vi "Do.vi"(8 "error in (no error)":errorcluster, 10 "Actor in":refnum<class "Actor.lvclass">, 11 "Update Fan Status Msg":refnum<class "Update Fan Status Msg.lvclass">) -> (0 "error out":errorcluster, 2 "Actor out":refnum<class "Actor.lvclass">)   [LabVIEW 2018, in "Evaporative Cooler Controller.lvlib" / "Update Fan Status Msg.lvclass"]
uses:
  Update Fan Status Msg.lvclass
  <vilib>/ActorFramework/Actor/Actor.lvclass
  Evaporative Cooler Controller/Evaporative Cooler Controller.lvclass
  C:/Program Files (x86)/National Instruments/LabVIEW 2018/vi.lib/ActorFramework/Actor/Actor.lvclass
  Update Fan Status Msg.lvclass/Update Fan Status Msg.ctl
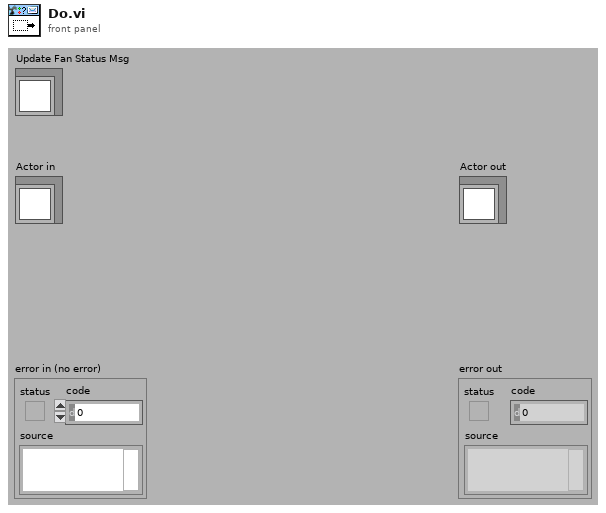
[diagram p1: front panel]
types:
  T1 = typedef "Dual Fan.lvlib/Dual Fan.lvclass/Fan Info.ctl" = cluster{"State":bool, "Fault":bool}
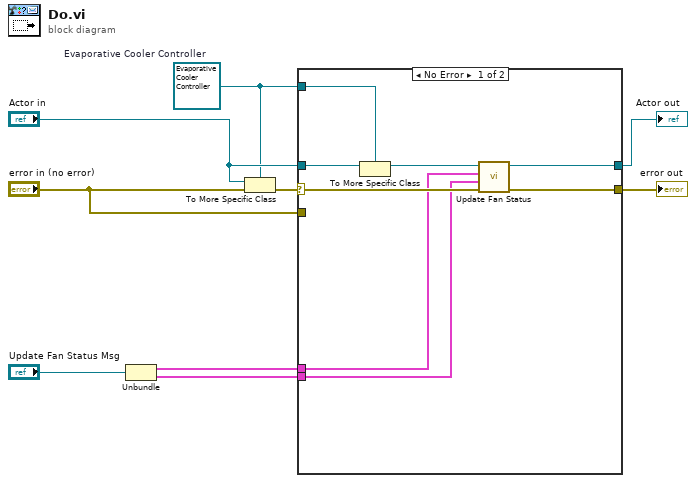
[diagram p0: block diagram]
diagram:
  w4 = refnum<class "Evaporative Cooler Controller.lvclass"> refnum  # Evaporative Cooler Controller
  n1 = Unbundle("Update Fan Status Msg") -> (w3:T1, w2:T1)
  n2 = To More Specific Class(target class=w4, reference="Actor in", error in="error in (no error)") -> (error out=w8:errorcluster)  [unwired: 1 out]
  n3 = case shown="No Error" w8 {
    selector: w8 -> [w15 _]
    tunnel: [w17 w18] -> w7
    tunnel: [w16 w19] -> w6
    tunnel: "Actor in" -> [w14 w19]
    tunnel: w4 -> [w13 _]
    tunnel: w3 -> [w11 _]
    tunnel: w2 -> [w10 _]
    tunnel: "error in (no error)" -> [_ w18]
    frame No Error {
      n4 = To More Specific Class(target class=w13, reference=w14) -> (specific class reference=w12:refnum<class "Evaporative Cooler Controller.lvclass">)  [unwired: 1 in, 1 out]
      n5 = call-dynamic "Update Fan Status.vi"("error in (no error)"=w15, "Fan B"=w10, "Fan A"=w11, "Evaporative Cooler Controller in"=w12) -> ("error out"=w17:errorcluster, "Evaporative Cooler Controller out"=w16:refnum<class "Evaporative Cooler Controller.lvclass">)  [unwired: 6 in]
    }
    frame Error {
      # "This Do.vi looks somewhat different from the standard. Here, we have decided that if this controller is not of the right type, that's ok. We ignore the error from the To More Specific Class function and just silently drop this message. This allows a plain Cooler Controller to control the Evaporative Cooler, even though a plain Cooler Controller has no idea how to handle all the messages coming out of the Evaporative Cooler. Since these are only status messages, we consider that to be ok."
    }
  }
  "error out" <- w7
  "Actor out" <- w6
